vi "Get Message Name.vi"(8 "error in (no error)":errorcluster, 11 "Message ref in":u64) -> (0 "error out":errorcluster, 1 "Message Name":string, 2 "Package Name":string, 3 "Message ref out":u64)   [LabVIEW 2019, in "gRPC Scripting Tools.lvlib"]
uses:
  gRPC Scripting Tools.lvlib
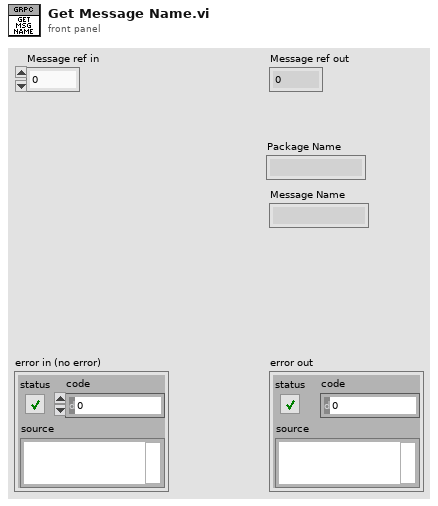
[diagram p1: front panel]
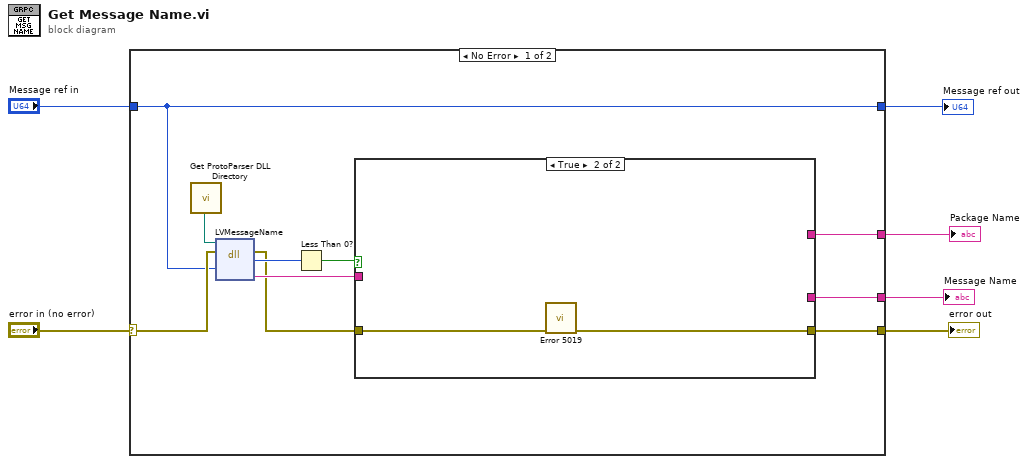
[diagram p0: block diagram]
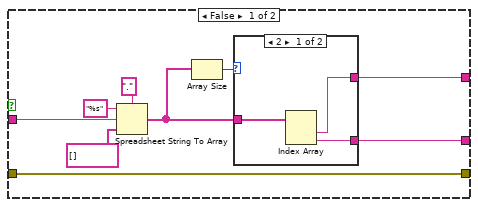
[diagram p2: hidden frame]
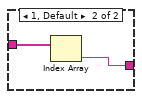
[diagram p3: hidden frame]
diagram:
  n1 = case shown="No Error" "error in (no error)" {
    selector: "error in (no error)" -> [w15 w34]
    tunnel: "Message ref in" -> [w14 w33]
    tunnel: [w14 w33] -> w4
    tunnel: [w7 w34] -> w3
    tunnel: [w12 _] -> w2
    tunnel: [w11 _] -> w1
    frame No Error {
      n2 = call "Get ProtoParser DLL Directory.vi"() -> ("Proto Parser Directory"=w16:path)
      n3 = dll-call lib="C:/Users/XEnderMD/Desktop/LV gRPC/labview source/gRPC Scripting Tools/Proto Parser API/dll/labview_grpc_generator.dll" fn="LVMessageName"(path in=w16, error in=w15, "message"=w14) -> (error out=w8:errorcluster, "return type"=w10:i32, "name"=w13:string)  [unwired: 3 in, 1 out]
      n4 = Less Than 0?(x=w10) -> (x < 0?=w9:bool)
      n5 = case shown="True" w9 {
        tunnel: w13 -> [w25 _]
        tunnel: [w19 _] -> w12
        tunnel: [w18 _] -> w11
        tunnel: w8 -> [w17 w32]
        tunnel: [w17 w31] -> w7
        frame False {
          n6 = Spreadsheet String To Array(delimiter (Tab)=".", format string="%s", spreadsheet string=w25, array type (2D Dbl)=string[] []) -> (array=w20:string[])
          n7 = Array Size(array=w20) -> (size(s)=w21:i32)
          n8 = case shown="2" w21 {
            tunnel: w20 -> [w28 w30]
            tunnel: [w27 w29] -> w19
            tunnel: [w26 _] -> w18
            frame 2 {
              n9 = Index Array(array=w28) -> (element #1=w26:string, element #2=w27:string)  [unwired: 2 in]
            }
            frame 1, Default {
              n10 = Index Array(array=w30) -> (element=w29:string)  [unwired: 1 in]
            }
          }
        }
        frame True {
          n11 = call "Error 5019.vi"("error in (no error)"=w32) -> ("error out"=w31:errorcluster)  [unwired: 10 in]
        }
      }
    }
    frame Error {
    }
  }
  "Message Name" <- w2
  "Message ref out" <- w4
  "error out" <- w3
  "Package Name" <- w1
